vi "Torque, Load, and Efficiency (Input Power).vi"(1 "additional efficiency information":T1(array[cluster]), 7 "speed [RPM]":dbl[](array[numeric]), 11 "error in (no error)":errorcluster, 12 "nameplate information":T2(array[cluster]), 13 "total input active power [W]":dbl[](array[numeric])) -> (4 "torque [Nm]":dbl[](array[numeric]), 6 "load [kW]":dbl[](array[numeric]), 8 "efficiency [%]":dbl[](array[numeric]), 15 "error out":errorcluster)   [LabVIEW 2014, in "NI_EP_Motor Monitoring.lvlib"]
doc: "Calculates the torque, load, and efficiency values based on the motor nameplate information. You must manually select the polymorphic instance you want to use."
uses:
  <vilib>/addons/Electrical Power/Motor Monitoring/NI_EP_Motor Monitoring.lvlib
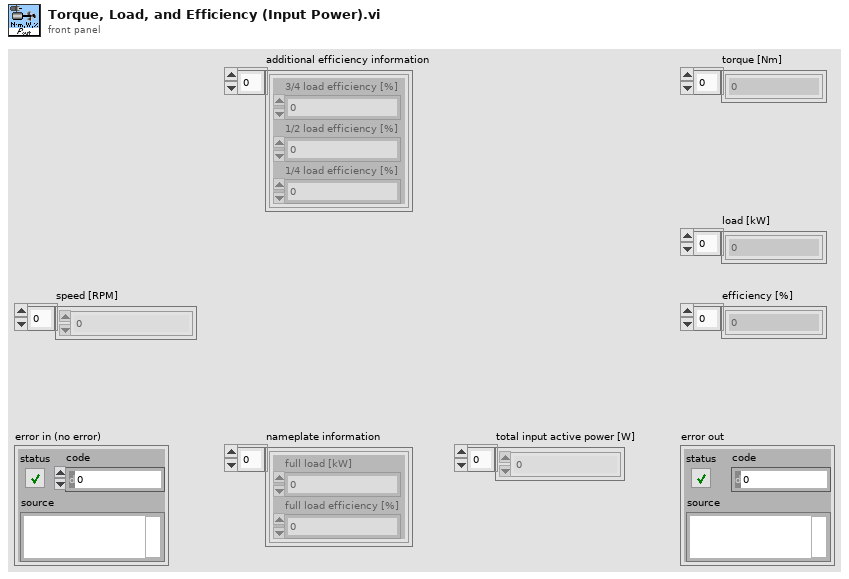
[diagram p1: front panel]
types:
  T1 = cluster{"3/4 load efficiency [%]":dbl, "1/2 load efficiency [%]":dbl, "1/4 load efficiency [%]":dbl}[]
  T2 = cluster{"full load [kW]":dbl, "full load efficiency [%]":dbl}[]
  T3 = cluster{"3/4 load efficiency [%]":dbl, "1/2 load efficiency [%]":dbl, "1/4 load efficiency [%]":dbl}
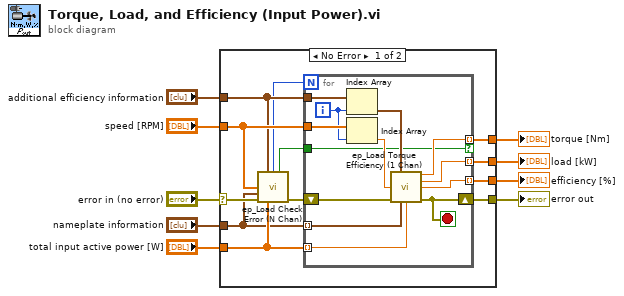
[diagram p0: block diagram]
diagram:
  n1 = case shown="No Error" "error in (no error)" {
    selector: "error in (no error)" -> [w21 w35]
    tunnel: [w19 w35] -> w8
    tunnel: "additional efficiency information" -> [w16 _]
    tunnel: "speed [RPM]" -> [w17 _]
    tunnel: "nameplate information" -> [w10 _]
    tunnel: "total input active power [W]" -> [w18 _]
    tunnel: [w15 _] -> w3
    tunnel: [w14 _] -> w2
    tunnel: [w13 _] -> w1
    frame No Error {
      n2 = call <vilib>:"ep_Load Check Error (N Chan).vi"("additional efficiency information"=w16, "speed [RPM]"=w17, "nameplate information"=w10, "error in (no error)"=w21, "total input active power [W]"=w18) -> ("number of motors"=w12:i32, "non-empty speed?"=w11:bool, "error out"=w20:errorcluster)  [unwired: 8 in]
      n3 = for {
        N: w12 -> [_]
        shift-right: [w32] -> w19
        shift-left: w20 -> [w34]
        tunnel: w18 -> [w23] mode=indexing
        tunnel: w17 -> [w27]
        tunnel: w16 -> [w28]
        tunnel: [w33] -> w15 mode=indexing
        tunnel: [w31] -> w14 mode=indexing
        tunnel: [w30] -> w13 mode=indexing if=w24
        tunnel: w11 -> [w24]
        tunnel: w10 -> [w22] mode=indexing
        i -> [w26]
        stop <- w32 stop-if-true
        n4 = Index Array(array=w28, index=w26) -> (element=w29:T3)
        n5 = Index Array(array=w27, index=w26) -> (element=w25:dbl)
        n6 = call <vilib>:"ep_Load Torque Efficiency (1 Chan).vi"("additional efficiency information"=w29, "speed [RPM]"=w25, "error in (no error)"=w34, "nameplate information"=w22, "total input active power [W]"=w23) -> ("torque [Nm]"=w30:dbl, "load [kW]"=w31:dbl, "efficiency [%]"=w33:dbl, "error out"=w32:errorcluster)  [unwired: 7 in]
      }
    }
    frame Error {
    }
  }
  "error out" <- w8
  "efficiency [%]" <- w3
  "torque [Nm]" <- w1
  "load [kW]" <- w2
